vi "Write GPU View.vi"(8 "error in (no error)":errorcluster, 10 "CPU View":T1 {"fwidth:" format="%#_6p"; "f0:" format="%#_6p"}, 11 "Simple UI in":refnum<class "Simple UI.lvclass">) -> (0 "error out":errorcluster, 3 "Simple UI out":refnum<class "Simple UI.lvclass">)   [LabVIEW 2020, in "Simple UI.lvlib" / "Simple UI.lvclass"]
uses:
  Simple UI.lvclass
  C:/Program Files/National Instruments/LabVIEW 2026/vi.lib/ActorFramework/Actor/Actor.lvclass
  chart zoom.ctl
  <vilib>/ActorFramework/Actor/Actor.lvclass/Actor.ctl
  Simple UI.lvclass/Simple UI.ctl
  Application Manager/Application Manager Messages/Set GPU View Msg/Set GPU View Msg.lvclass/Set GPU View Msg.ctl
  <vilib>/ActorFramework/Message Enqueuer/Message Enqueuer.lvclass/Message Enqueuer.ctl
  <vilib>/ActorFramework/Message Enqueuer/Enqueue.vi
  Application Manager/Application Manager Messages/Set GPU View Msg/Set GPU View Msg.lvclass
  C:/Program Files/National Instruments/LabVIEW 2026/vi.lib/ActorFramework/Message/Message.lvclass
  <vilib>/ActorFramework/Message Priority Queue/Priority Enqueue.vi
  <vilib>/ActorFramework/Actor/Actor.lvclass
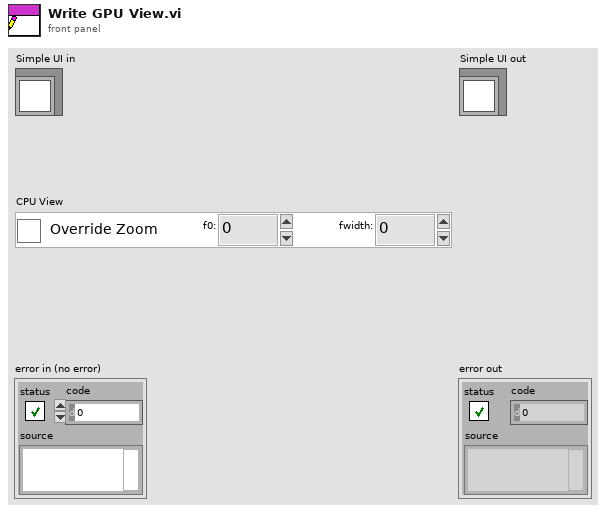
[diagram p1: front panel]
types:
  T1 = typedef "Simple UI.lvlib/Simple UI.lvclass/chart zoom.ctl" = cluster{"Override":bool, "f0: ":dbl, "fwidth: ":dbl}
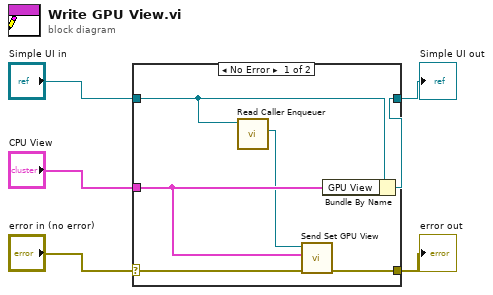
[diagram p0: block diagram]
diagram:
  n1 = case shown="No Error" "error in (no error)" {
    selector: "error in (no error)" -> [w10 w12]
    tunnel: [w9 w12] -> w4
    tunnel: [w11 w13] -> w2
    tunnel: "Simple UI in" -> [w7 w13]
    tunnel: "CPU View" -> [w8 _]
    frame No Error {
      n2 = call <vilib>:"Read Caller Enqueuer.vi"("Actor"=w7) -> ("Caller Enqueuer"=w6:refnum<class "Message Enqueuer.lvclass">)  [unwired: 10 in]
      n3 = call "Send Set GPU View.vi"("error in (no error)"=w10, "GPU View"=w8, "Message Enqueuer"=w6) -> ("error out"=w9:errorcluster)  [unwired: 7 in, 1 out]
      n4 = Bundle By Name(cluster=w7, "GPU View"=w8) -> (w11:refnum<class "Simple UI.lvclass">)
    }
    frame Error {
    }
  }
  "error out" <- w4
  "Simple UI out" <- w2
